vi "TryUpdateDisplacementSample.vi"   [LabVIEW 2016]
uses:
  <vilib>/rvi/DataTransferAndStorage/Container/XNode/niFpgaContainer.xnode
  <vilib>/rvi/FIFO/Fifo_Resource/nirvififoEmulationRead.vi
  <vilib>/rvi/FIFO/Fifo_Resource/nirvififoEmulationWrite.vi
  Telemetry/TelemetryDataTypes.ctl
  Telemetry/TelemetryUpdateModes.ctl
  Telemetry/TelemetryFields.ctl
  <vilib>/rvi/DataTransferAndStorage/Register/Emulation/niFpgaRegisterEmulation.vi
  <vilib>/Platform/TimedLoop/XDataNode/XDataNode.xnode
  <vilib>/Platform/TimedLoop/XDataNode/nitl_modes.ctl
  <vilib>/Platform/TimedLoop/XDataNode/XDNodeRunTimeDep.lvlib
  <vilib>/Platform/TimedLoop/XDataNode/wakeup.ctl
  <vilib>/Platform/TimedLoop/XDataNode/timing_clust.ctl
types:
  T1 = cluster{"Timestamp":u64, "TxBytes":u64, "RxBytes":u64, "TxFrames":u64, "RxFrames":u64, "Sensor1Raw":i32, "Sensor2Raw":i32, "Sensor3Raw":i32, "Sensor4Raw":i32, "Sensor5Raw":i32, "Sensor6Raw":i32, "Sensor7Raw":i32, "Sensor8Raw":i32, "Sensor1Eng":sgl, "Sensor2Eng":sgl, "Sensor3Eng":sgl, "Sensor4Eng":sgl, "Sensor5Eng":sgl, "Sensor6Eng":sgl, "Sensor7Eng":sgl, "Sensor8Eng":sgl, "PositionX":sgl, "PositionY":sgl, "PositionZ":sgl, "RotationX":sgl, "RotationY":sgl, "RotationZ":sgl}
  T2 = typedef "TelemetryFields.ctl" = enum16{"None", "InclinometerTxBytes", "InclinometerRxBytes", "InclinometerTxFrames", "InclinometerRxFrames", "InclinometerErrorTimestamp", "InclinometerErrorCode", "InclinometerSampleTimestamp", "InclinometerRawAngle", "InclinometerZenithAngle", "DisplacementTxBytes", "DisplacementRxBytes", "DisplacementTxFrames", "DisplacementRxFrames", "DisplacementErrorTimestamp", "DisplacementErrorCode", "DisplacementSampleTimestamp", "DisplacementRaw1", "DisplacementRaw2", "DisplacementRaw3", "DisplacementRaw4", "DisplacementRaw5", "DisplacementRaw6", "DisplacementRaw7", "DisplacementRaw8", "DisplacementEng1", "DisplacementEng2", "DisplacementEng3", "DisplacementEng4", "DisplacementEng5", "DisplacementEng6", "DisplacementEng7", "DisplacementEng8", "DisplacementPositionX", "DisplacementPositionY", "DisplacementPositionZ", "DisplacementRotationX", "DisplacementRotationY", "DisplacementRotationZ", "AccelerometerSampleCount", "AccelerometerSampleTimestamp", "AccelerometerRaw1", "AccelerometerRaw2", "AccelerometerRaw3", "AccelerometerRaw4", "AccelerometerRaw5", "AccelerometerRaw6", "AccelerometerRaw7", "AccelerometerRaw8", "AccelerometerEng1", "AccelerometerEng2", "AccelerometerEng3", "AccelerometerEng4", "AccelerometerEng5", "AccelerometerEng6", "AccelerometerEng7", "AccelerometerEng8", "AngularAccelerationX", "AngularAccelerationY", "AngularAccelerationZ", "GyroTxBytes", "GyroRxBytes", "GyroTxFrames", "GyroRxFrames", "GyroErrorTimestamp", "GyroErrorCode", "GyroSampleTimestamp", "GyroX", "GyroY", "GyroZ", "GyroStatus", "GyroSequenceNumber", "GyroTemperature", "GyroBITTimestamp", "GyroBIT0", "GyroBIT1", "GyroBIT2", "GyroBIT3", "GyroBIT4", "GyroBIT5", "GyroBIT6", "GyroBIT7"}
  T3 = typedef "TelemetryUpdateModes.ctl" = enum8{"=", "+", "-", "|"}
  T4 = typedef "TelemetryDataTypes.ctl" = enum8{"U8", "U16", "U32", "U64", "I8", "I16", "I32", "I64", "SGL"}
  T5 = typedef "XDNodeRunTimeDep.lvlib/timing_clust.ctl" = cluster{"Expected End [f-1]":u64, "Actual End [f-1]":u64, "Finished Late? [f-1]":bool, "Expected End [i-1]":u64, "Actual End [i-1]":u64, "Finished Late? [i-1]":bool, "Expected Start [i]":u64, "Actual Start [i]":u64, "Expected Start [f]":u64, "Actual Start [f]":u64, "Source Name":string, "Structure Name":string, "Period":i64, "Deadline":i64, "Offset":i64, "Start":i64, "Priority":i32, "Timeout":i32, "Mode":T6, "Wakeup Reason":T7, "Error":errorcluster, "Source Type":string, "Secondary Source Type":string, "Global End Time":u64, "Global Start Time":u64, "Frame Duration":u64, "Iteration Duration":u64, "Assigned CPU":i32, "I/O Scan Engine Mode":u32}
  T6 = typedef "XDNodeRunTimeDep.lvlib/nitl_modes.ctl" = enum32{"No Change", "Process missed periods, maintain original phase", "Discard missed periods, maintain original phase", "Process missed periods, ignore original phase", "Discard missed periods, ignore original phase"}
  T7 = typedef "XDNodeRunTimeDep.lvlib/wakeup.ctl" = enum32{"Normal", "Aborted", "Asynchronous wakeup", "Timing source error", "Timed loop error", "Timeout"}
  T8 = typedef "TelemetryUpdateData.ctl" = cluster{"DataType":T4, "Mode":T3, "Field":T2, "Data":u64}
  T9 = typedef "TelemetryUpdateDataSGL.ctl" = cluster{"Mode":T3, "Field":T2, "Data":sgl}
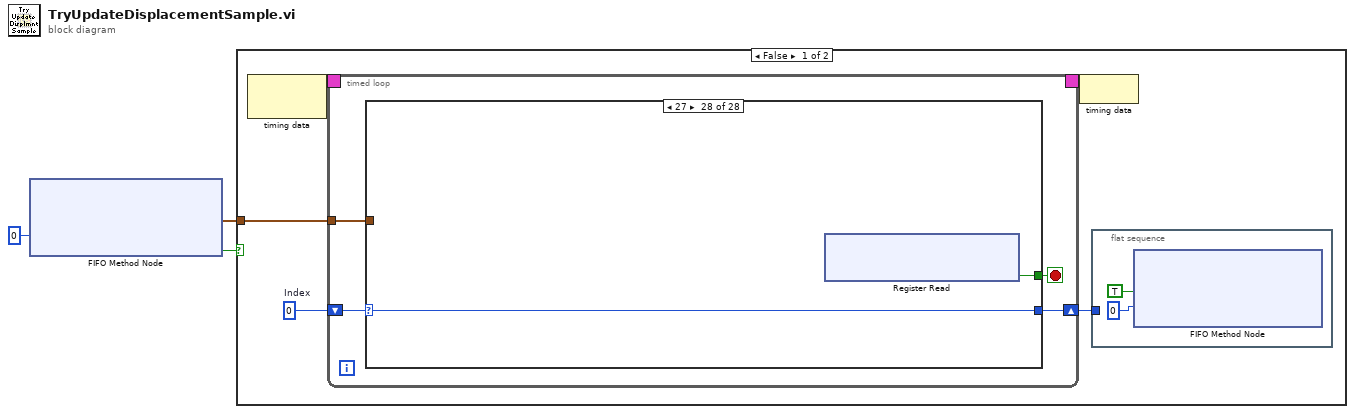
[diagram p0: block diagram]
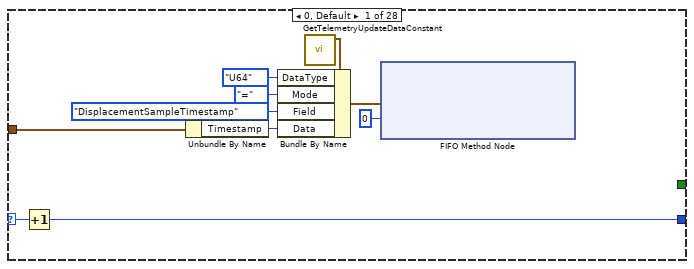
[diagram p2: hidden frame]
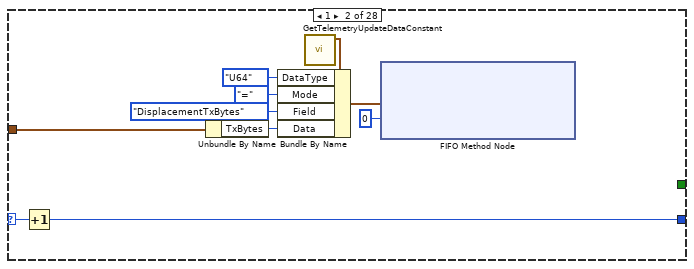
[diagram p3: hidden frame]
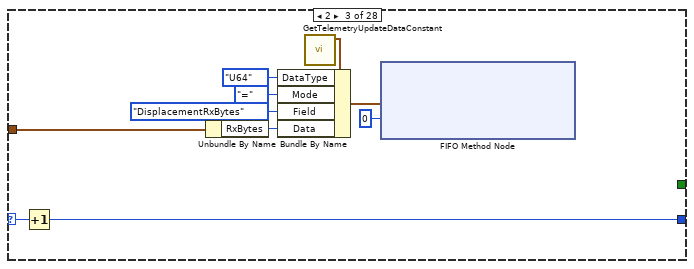
[diagram p4: hidden frame]
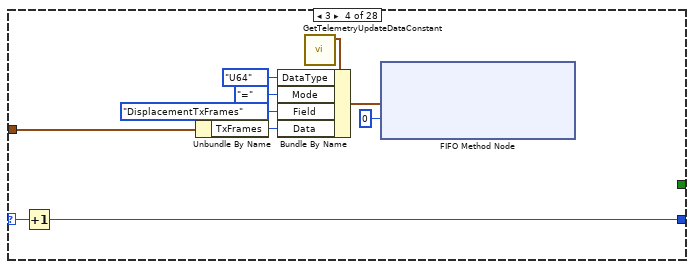
[diagram p5: hidden frame]
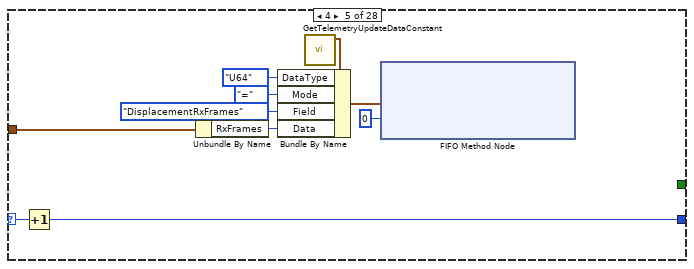
[diagram p6: hidden frame]
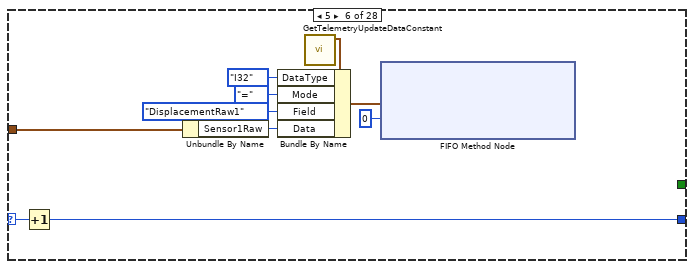
[diagram p7: hidden frame]
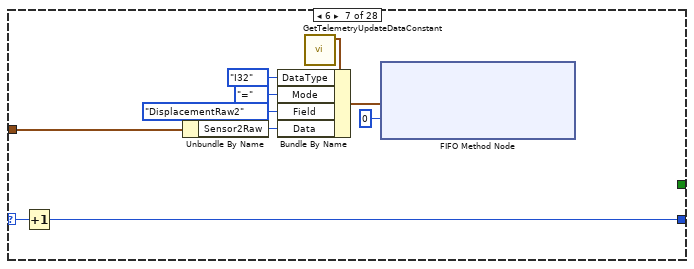
[diagram p8: hidden frame]
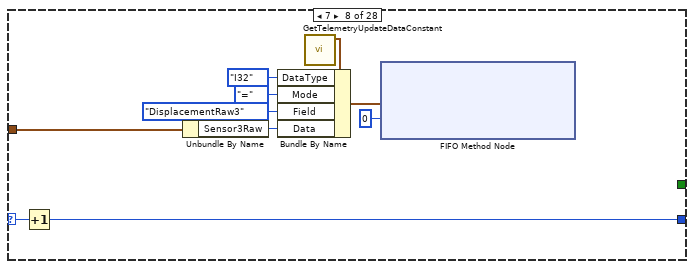
[diagram p9: hidden frame]
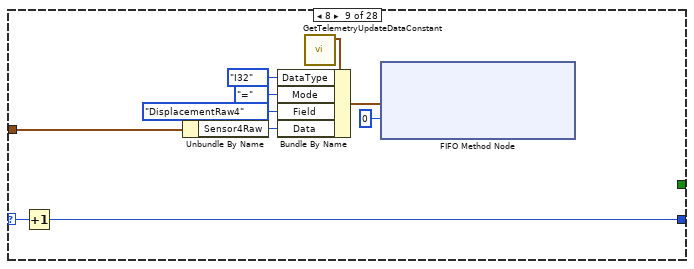
[diagram p10: hidden frame]
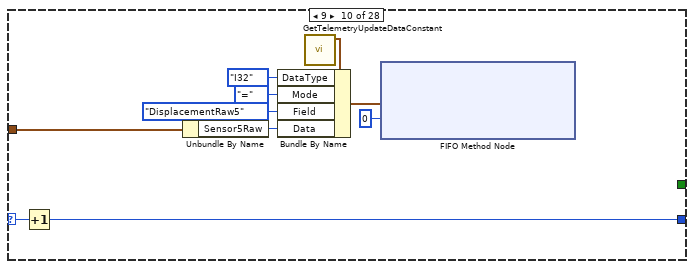
[diagram p11: hidden frame]
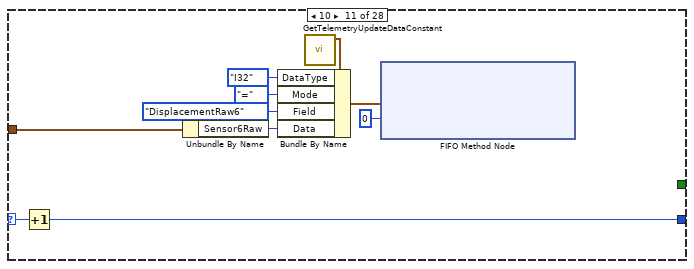
[diagram p12: hidden frame]
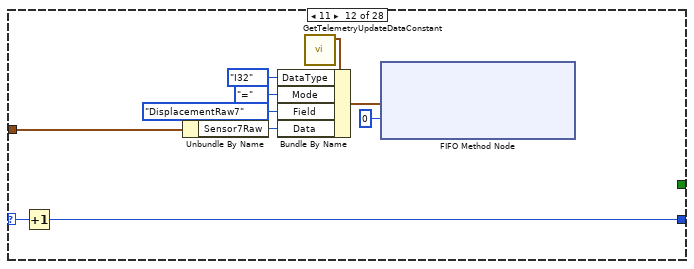
[diagram p13: hidden frame]
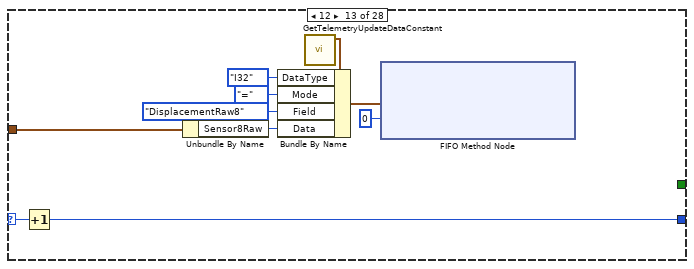
[diagram p14: hidden frame]
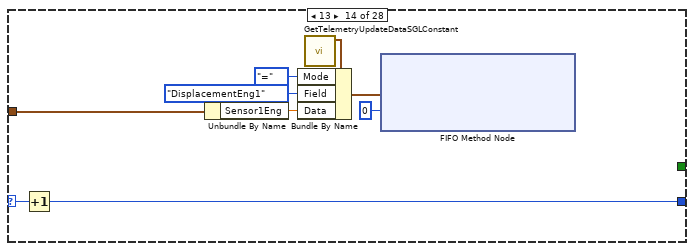
[diagram p15: hidden frame]
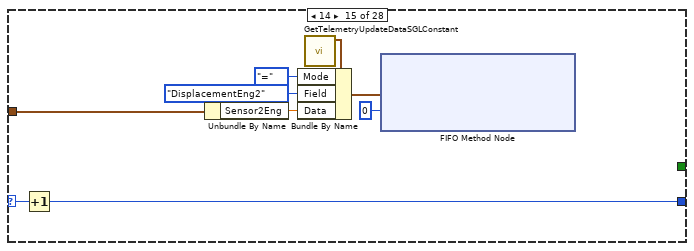
[diagram p16: hidden frame]
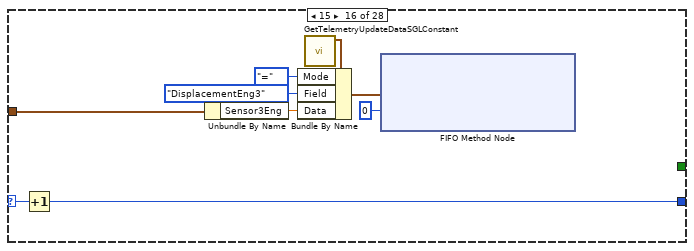
[diagram p17: hidden frame]
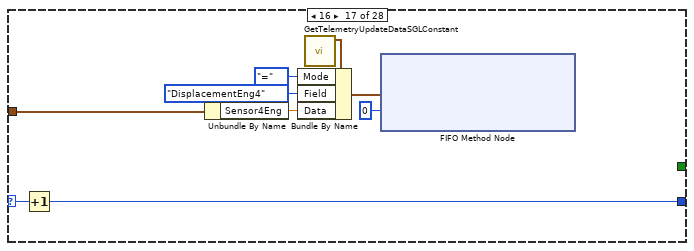
[diagram p18: hidden frame]
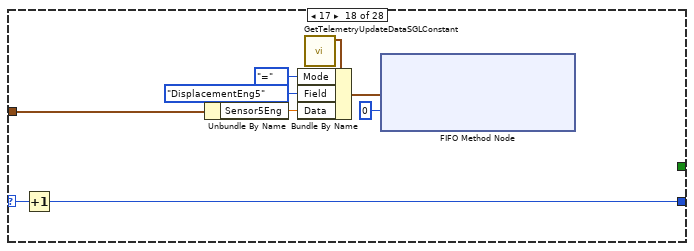
[diagram p19: hidden frame]
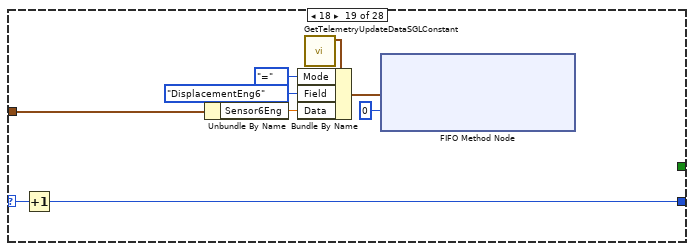
[diagram p20: hidden frame]
diagram:
  n1 = xnode ("FIFO Method Node")("Timeout"=0) -> ("Element"=w1:T1, "Timed Out?"=w2:bool)  [unwired: 1 in, 1 out]
  n2 = case shown="False" w2 {
    tunnel: w1 -> [w7 _]
    frame False {
      w8 = u8 0  # Index
      n3 = node-c288() -> (w5:T5)  [unwired: 1 in]
      n4 = timed-loop {
        shift-right: [w11] -> w6
        shift-left: w8 -> [w12]
        tunnel: w7 -> [w10]
        timing: w5 -> [_]
        timing-out: [_] -> w4
        stop <- w9 stop-if-true
        n5 = case shown="27" w12 {
          selector: w12 -> [w22 w32 w42 w52 w62 w72 w82 w92 w102 w112 w122 w132 w142 w151 w160 w169 w178 w187 w196 w205 w214 w223 w232 w241 w250 w259 w268 w270]
          tunnel: [w21 w31 w41 w51 w61 w71 w81 w91 w101 w111 w121 w131 w141 w150 w159 w168 w177 w186 w195 w204 w213 w222 w231 w240 w249 w258 w267 w270] -> w11
          tunnel: w10 -> [w13 w23 w33 w43 w53 w63 w73 w83 w93 w103 w113 w123 w133 w143 w152 w161 w170 w179 w188 w197 w206 w215 w224 w233 w242 w251 w260 _]
          tunnel: [_ _ _ _ _ _ _ _ _ _ _ _ _ _ _ _ _ _ _ _ _ _ _ _ _ _ _ w269] -> w9
          frame 0, Default {
            n6 = Increment(x=w22) -> (x+1=w21:u8)
            n7 = Unbundle By Name(w13) -> ("Timestamp"=w19:u64)
            n8 = call "GetTelemetryUpdateDataConstant.vi"() -> ("TelemetryUpdateData"=w18:T8)  [unwired: 11 in]
            n9 = Bundle By Name(cluster=w18, "DataType"=TelemetryDataTypes."U64", "Mode"=TelemetryUpdateModes."=", "Field"=TelemetryFields."DisplacementSampleTimestamp" ("TelemetryFields"), "Data"=w19) -> (w15:T8)
            n10 = xnode ("FIFO Method Node")("Element"=w15, "Timeout"=0) -> ()  [unwired: 1 in, 2 out]
          }
          frame 1 {
            n11 = Increment(x=w32) -> (x+1=w31:u8)
            n12 = Unbundle By Name(w23) -> ("TxBytes"=w24:u64)
            n13 = call "GetTelemetryUpdateDataConstant.vi"() -> ("TelemetryUpdateData"=w25:T8)  [unwired: 11 in]
            n14 = Bundle By Name(cluster=w25, "DataType"=TelemetryDataTypes."U64", "Mode"=TelemetryUpdateModes."=", "Field"=TelemetryFields."DisplacementTxBytes", "Data"=w24) -> (w29:T8)
            n15 = xnode ("FIFO Method Node")("Element"=w29, "Timeout"=0) -> ()  [unwired: 1 in, 2 out]
          }
          frame 2 {
            n16 = Increment(x=w42) -> (x+1=w41:u8)
            n17 = Unbundle By Name(w33) -> ("RxBytes"=w40:u64)
            n18 = call "GetTelemetryUpdateDataConstant.vi"() -> ("TelemetryUpdateData"=w39:T8)  [unwired: 11 in]
            n19 = Bundle By Name(cluster=w39, "DataType"=TelemetryDataTypes."U64", "Mode"=TelemetryUpdateModes."=", "Field"=TelemetryFields."DisplacementRxBytes", "Data"=w40) -> (w35:T8)
            n20 = xnode ("FIFO Method Node")("Element"=w35, "Timeout"=0) -> ()  [unwired: 1 in, 2 out]
          }
          frame 3 {
            n21 = Increment(x=w52) -> (x+1=w51:u8)
            n22 = Unbundle By Name(w43) -> ("TxFrames"=w44:u64)
            n23 = call "GetTelemetryUpdateDataConstant.vi"() -> ("TelemetryUpdateData"=w45:T8)  [unwired: 11 in]
            n24 = Bundle By Name(cluster=w45, "DataType"=TelemetryDataTypes."U64", "Mode"=TelemetryUpdateModes."=", "Field"=TelemetryFields."DisplacementTxFrames", "Data"=w44) -> (w49:T8)
            n25 = xnode ("FIFO Method Node")("Element"=w49, "Timeout"=0) -> ()  [unwired: 1 in, 2 out]
          }
          frame 4 {
            n26 = Increment(x=w62) -> (x+1=w61:u8)
            n27 = Unbundle By Name(w53) -> ("RxFrames"=w60:u64)
            n28 = call "GetTelemetryUpdateDataConstant.vi"() -> ("TelemetryUpdateData"=w59:T8)  [unwired: 11 in]
            n29 = Bundle By Name(cluster=w59, "DataType"=TelemetryDataTypes."U64", "Mode"=TelemetryUpdateModes."=", "Field"=TelemetryFields."DisplacementRxFrames", "Data"=w60) -> (w55:T8)
            n30 = xnode ("FIFO Method Node")("Element"=w55, "Timeout"=0) -> ()  [unwired: 1 in, 2 out]
          }
          frame 5 {
            n31 = Increment(x=w72) -> (x+1=w71:u8)
            n32 = Unbundle By Name(w63) -> ("Sensor1Raw"=w64:i32)
            n33 = call "GetTelemetryUpdateDataConstant.vi"() -> ("TelemetryUpdateData"=w65:T8)  [unwired: 11 in]
            n34 = Bundle By Name(cluster=w65, "DataType"=TelemetryDataTypes."I32", "Mode"=TelemetryUpdateModes."=", "Field"=TelemetryFields."DisplacementRaw1" ("TelemetryFields"), "Data"=w64) -> (w68:T8)
            n35 = xnode ("FIFO Method Node")("Element"=w68, "Timeout"=0) -> ()  [unwired: 1 in, 2 out]
          }
          frame 6 {
            n36 = Increment(x=w82) -> (x+1=w81:u8)
            n37 = Unbundle By Name(w73) -> ("Sensor2Raw"=w79:i32)
            n38 = call "GetTelemetryUpdateDataConstant.vi"() -> ("TelemetryUpdateData"=w78:T8)  [unwired: 11 in]
            n39 = Bundle By Name(cluster=w78, "DataType"=TelemetryDataTypes."I32", "Mode"=TelemetryUpdateModes."=", "Field"=TelemetryFields."DisplacementRaw2" ("TelemetryFields"), "Data"=w79) -> (w75:T8)
            n40 = xnode ("FIFO Method Node")("Element"=w75, "Timeout"=0) -> ()  [unwired: 1 in, 2 out]
          }
          frame 7 {
            n41 = Increment(x=w92) -> (x+1=w91:u8)
            n42 = Unbundle By Name(w83) -> ("Sensor3Raw"=w84:i32)
            n43 = call "GetTelemetryUpdateDataConstant.vi"() -> ("TelemetryUpdateData"=w85:T8)  [unwired: 11 in]
            n44 = Bundle By Name(cluster=w85, "DataType"=TelemetryDataTypes."I32", "Mode"=TelemetryUpdateModes."=", "Field"=TelemetryFields."DisplacementRaw3" ("TelemetryFields"), "Data"=w84) -> (w88:T8)
            n45 = xnode ("FIFO Method Node")("Element"=w88, "Timeout"=0) -> ()  [unwired: 1 in, 2 out]
          }
          frame 8 {
            n46 = Increment(x=w102) -> (x+1=w101:u8)
            n47 = Unbundle By Name(w93) -> ("Sensor4Raw"=w99:i32)
            n48 = call "GetTelemetryUpdateDataConstant.vi"() -> ("TelemetryUpdateData"=w98:T8)  [unwired: 11 in]
            n49 = Bundle By Name(cluster=w98, "DataType"=TelemetryDataTypes."I32", "Mode"=TelemetryUpdateModes."=", "Field"=TelemetryFields."DisplacementRaw4" ("TelemetryFields"), "Data"=w99) -> (w95:T8)
            n50 = xnode ("FIFO Method Node")("Element"=w95, "Timeout"=0) -> ()  [unwired: 1 in, 2 out]
          }
          frame 9 {
            n51 = Increment(x=w112) -> (x+1=w111:u8)
            n52 = Unbundle By Name(w103) -> ("Sensor5Raw"=w104:i32)
            n53 = call "GetTelemetryUpdateDataConstant.vi"() -> ("TelemetryUpdateData"=w105:T8)  [unwired: 11 in]
            n54 = Bundle By Name(cluster=w105, "DataType"=TelemetryDataTypes."I32", "Mode"=TelemetryUpdateModes."=", "Field"=TelemetryFields."DisplacementRaw5" ("TelemetryFields"), "Data"=w104) -> (w108:T8)
            n55 = xnode ("FIFO Method Node")("Element"=w108, "Timeout"=0) -> ()  [unwired: 1 in, 2 out]
          }
          frame 10 {
            n56 = Increment(x=w122) -> (x+1=w121:u8)
            n57 = Unbundle By Name(w113) -> ("Sensor6Raw"=w119:i32)
            n58 = call "GetTelemetryUpdateDataConstant.vi"() -> ("TelemetryUpdateData"=w118:T8)  [unwired: 11 in]
            n59 = Bundle By Name(cluster=w118, "DataType"=TelemetryDataTypes."I32", "Mode"=TelemetryUpdateModes."=", "Field"=TelemetryFields."DisplacementRaw6" ("TelemetryFields"), "Data"=w119) -> (w115:T8)
            n60 = xnode ("FIFO Method Node")("Element"=w115, "Timeout"=0) -> ()  [unwired: 1 in, 2 out]
          }
          frame 11 {
            n61 = Increment(x=w132) -> (x+1=w131:u8)
            n62 = Unbundle By Name(w123) -> ("Sensor7Raw"=w124:i32)
            n63 = call "GetTelemetryUpdateDataConstant.vi"() -> ("TelemetryUpdateData"=w125:T8)  [unwired: 11 in]
            n64 = Bundle By Name(cluster=w125, "DataType"=TelemetryDataTypes."I32", "Mode"=TelemetryUpdateModes."=", "Field"=TelemetryFields."DisplacementRaw7" ("TelemetryFields"), "Data"=w124) -> (w128:T8)
            n65 = xnode ("FIFO Method Node")("Element"=w128, "Timeout"=0) -> ()  [unwired: 1 in, 2 out]
          }
          frame 12 {
            n66 = Increment(x=w142) -> (x+1=w141:u8)
            n67 = Unbundle By Name(w133) -> ("Sensor8Raw"=w139:i32)
            n68 = call "GetTelemetryUpdateDataConstant.vi"() -> ("TelemetryUpdateData"=w138:T8)  [unwired: 11 in]
            n69 = Bundle By Name(cluster=w138, "DataType"=TelemetryDataTypes."I32", "Mode"=TelemetryUpdateModes."=", "Field"=TelemetryFields."DisplacementRaw8" ("TelemetryFields"), "Data"=w139) -> (w135:T8)
            n70 = xnode ("FIFO Method Node")("Element"=w135, "Timeout"=0) -> ()  [unwired: 1 in, 2 out]
          }
          frame 13 {
            n71 = Increment(x=w151) -> (x+1=w150:u8)
            n72 = Unbundle By Name(w143) -> ("Sensor1Eng"=w149:sgl)
            n73 = call "GetTelemetryUpdateDataSGLConstant.vi"() -> ("TelemetryUpdateDataSGL"=w144:T9)  [unwired: 11 in]
            n74 = Bundle By Name(cluster=w144, "Mode"=TelemetryUpdateModes."=", "Field"=TelemetryFields."DisplacementEng1", "Data"=w149) -> (w145:T9)
            n75 = xnode ("FIFO Method Node")("Element"=w145, "Timeout"=0) -> ()  [unwired: 1 in, 2 out]
          }
          frame 14 {
            n76 = Increment(x=w160) -> (x+1=w159:u8)
            n77 = Unbundle By Name(w152) -> ("Sensor2Eng"=w158:sgl)
            n78 = call "GetTelemetryUpdateDataSGLConstant.vi"() -> ("TelemetryUpdateDataSGL"=w153:T9)  [unwired: 11 in]
            n79 = Bundle By Name(cluster=w153, "Mode"=TelemetryUpdateModes."=", "Field"=TelemetryFields."DisplacementEng2", "Data"=w158) -> (w154:T9)
            n80 = xnode ("FIFO Method Node")("Element"=w154, "Timeout"=0) -> ()  [unwired: 1 in, 2 out]
          }
          frame 15 {
            n81 = Increment(x=w169) -> (x+1=w168:u8)
            n82 = Unbundle By Name(w161) -> ("Sensor3Eng"=w167:sgl)
            n83 = call "GetTelemetryUpdateDataSGLConstant.vi"() -> ("TelemetryUpdateDataSGL"=w162:T9)  [unwired: 11 in]
            n84 = Bundle By Name(cluster=w162, "Mode"=TelemetryUpdateModes."=", "Field"=TelemetryFields."DisplacementEng3", "Data"=w167) -> (w163:T9)
            n85 = xnode ("FIFO Method Node")("Element"=w163, "Timeout"=0) -> ()  [unwired: 1 in, 2 out]
          }
          frame 16 {
            n86 = Increment(x=w178) -> (x+1=w177:u8)
            n87 = Unbundle By Name(w170) -> ("Sensor4Eng"=w176:sgl)
            n88 = call "GetTelemetryUpdateDataSGLConstant.vi"() -> ("TelemetryUpdateDataSGL"=w171:T9)  [unwired: 11 in]
            n89 = Bundle By Name(cluster=w171, "Mode"=TelemetryUpdateModes."=", "Field"=TelemetryFields."DisplacementEng4", "Data"=w176) -> (w172:T9)
            n90 = xnode ("FIFO Method Node")("Element"=w172, "Timeout"=0) -> ()  [unwired: 1 in, 2 out]
          }
          frame 17 {
            n91 = Increment(x=w187) -> (x+1=w186:u8)
            n92 = Unbundle By Name(w179) -> ("Sensor5Eng"=w185:sgl)
            n93 = call "GetTelemetryUpdateDataSGLConstant.vi"() -> ("TelemetryUpdateDataSGL"=w180:T9)  [unwired: 11 in]
            n94 = Bundle By Name(cluster=w180, "Mode"=TelemetryUpdateModes."=", "Field"=TelemetryFields."DisplacementEng5", "Data"=w185) -> (w181:T9)
            n95 = xnode ("FIFO Method Node")("Element"=w181, "Timeout"=0) -> ()  [unwired: 1 in, 2 out]
          }
          frame 18 {
            n96 = Increment(x=w196) -> (x+1=w195:u8)
            n97 = Unbundle By Name(w188) -> ("Sensor6Eng"=w194:sgl)
            n98 = call "GetTelemetryUpdateDataSGLConstant.vi"() -> ("TelemetryUpdateDataSGL"=w189:T9)  [unwired: 11 in]
            n99 = Bundle By Name(cluster=w189, "Mode"=TelemetryUpdateModes."=", "Field"=TelemetryFields."DisplacementEng6", "Data"=w194) -> (w190:T9)
            n100 = xnode ("FIFO Method Node")("Element"=w190, "Timeout"=0) -> ()  [unwired: 1 in, 2 out]
          }
          frame 19 {
            n101 = Increment(x=w205) -> (x+1=w204:u8)
            n102 = Unbundle By Name(w197) -> ("Sensor7Eng"=w203:sgl)
            n103 = call "GetTelemetryUpdateDataSGLConstant.vi"() -> ("TelemetryUpdateDataSGL"=w198:T9)  [unwired: 11 in]
            n104 = Bundle By Name(cluster=w198, "Mode"=TelemetryUpdateModes."=", "Field"=TelemetryFields."DisplacementEng7", "Data"=w203) -> (w199:T9)
            n105 = xnode ("FIFO Method Node")("Element"=w199, "Timeout"=0) -> ()  [unwired: 1 in, 2 out]
          }
          frame 20 {
            n106 = Increment(x=w214) -> (x+1=w213:u8)
            n107 = Unbundle By Name(w206) -> ("Sensor8Eng"=w212:sgl)
            n108 = call "GetTelemetryUpdateDataSGLConstant.vi"() -> ("TelemetryUpdateDataSGL"=w207:T9)  [unwired: 11 in]
            n109 = Bundle By Name(cluster=w207, "Mode"=TelemetryUpdateModes."=", "Field"=TelemetryFields."DisplacementEng8", "Data"=w212) -> (w208:T9)
            n110 = xnode ("FIFO Method Node")("Element"=w208, "Timeout"=0) -> ()  [unwired: 1 in, 2 out]
          }
          frame 21 {
            n111 = Increment(x=w223) -> (x+1=w222:u8)
            n112 = Unbundle By Name(w215) -> ("PositionX"=w221:sgl)
            n113 = call "GetTelemetryUpdateDataSGLConstant.vi"() -> ("TelemetryUpdateDataSGL"=w216:T9)  [unwired: 11 in]
            n114 = Bundle By Name(cluster=w216, "Mode"=TelemetryUpdateModes."=", "Field"=TelemetryFields."DisplacementPositionX", "Data"=w221) -> (w217:T9)
            n115 = xnode ("FIFO Method Node")("Element"=w217, "Timeout"=0) -> ()  [unwired: 1 in, 2 out]
          }
          frame 22 {
            n116 = Increment(x=w232) -> (x+1=w231:u8)
            n117 = Unbundle By Name(w224) -> ("PositionY"=w230:sgl)
            n118 = call "GetTelemetryUpdateDataSGLConstant.vi"() -> ("TelemetryUpdateDataSGL"=w225:T9)  [unwired: 11 in]
            n119 = Bundle By Name(cluster=w225, "Mode"=TelemetryUpdateModes."=", "Field"=TelemetryFields."DisplacementPositionY", "Data"=w230) -> (w226:T9)
            n120 = xnode ("FIFO Method Node")("Element"=w226, "Timeout"=0) -> ()  [unwired: 1 in, 2 out]
          }
          frame 23 {
            n121 = Increment(x=w241) -> (x+1=w240:u8)
            n122 = Unbundle By Name(w233) -> ("PositionZ"=w239:sgl)
            n123 = call "GetTelemetryUpdateDataSGLConstant.vi"() -> ("TelemetryUpdateDataSGL"=w234:T9)  [unwired: 11 in]
            n124 = Bundle By Name(cluster=w234, "Mode"=TelemetryUpdateModes."=", "Field"=TelemetryFields."DisplacementPositionZ", "Data"=w239) -> (w235:T9)
            n125 = xnode ("FIFO Method Node")("Element"=w235, "Timeout"=0) -> ()  [unwired: 1 in, 2 out]
          }
          frame 24 {
            n126 = Increment(x=w250) -> (x+1=w249:u8)
            n127 = Unbundle By Name(w242) -> ("RotationX"=w248:sgl)
            n128 = call "GetTelemetryUpdateDataSGLConstant.vi"() -> ("TelemetryUpdateDataSGL"=w243:T9)  [unwired: 11 in]
            n129 = Bundle By Name(cluster=w243, "Mode"=TelemetryUpdateModes."=", "Field"=TelemetryFields."DisplacementRotationX", "Data"=w248) -> (w244:T9)
            n130 = xnode ("FIFO Method Node")("Element"=w244, "Timeout"=0) -> ()  [unwired: 1 in, 2 out]
          }
          frame 25 {
            n131 = Increment(x=w259) -> (x+1=w258:u8)
            n132 = Unbundle By Name(w251) -> ("RotationY"=w257:sgl)
            n133 = call "GetTelemetryUpdateDataSGLConstant.vi"() -> ("TelemetryUpdateDataSGL"=w252:T9)  [unwired: 11 in]
            n134 = Bundle By Name(cluster=w252, "Mode"=TelemetryUpdateModes."=", "Field"=TelemetryFields."DisplacementRotationY", "Data"=w257) -> (w253:T9)
            n135 = xnode ("FIFO Method Node")("Element"=w253, "Timeout"=0) -> ()  [unwired: 1 in, 2 out]
          }
          frame 26 {
            n136 = Increment(x=w268) -> (x+1=w267:u8)
            n137 = Unbundle By Name(w260) -> ("RotationZ"=w266:sgl)
            n138 = call "GetTelemetryUpdateDataSGLConstant.vi"() -> ("TelemetryUpdateDataSGL"=w261:T9)  [unwired: 11 in]
            n139 = Bundle By Name(cluster=w261, "Mode"=TelemetryUpdateModes."=", "Field"=TelemetryFields."DisplacementRotationZ", "Data"=w266) -> (w262:T9)
            n140 = xnode ("FIFO Method Node")("Element"=w262, "Timeout"=0) -> ()  [unwired: 1 in, 2 out]
          }
          frame 27 {
            n141 = xnode ("Register Read")() -> ("Data"=w269:bool)  [unwired: 1 in, 1 out]
          }
        }
      }
      n142 = node-c288(w4) -> ()
      n143 = flat-sequence {
        tunnel: w6 -> [_]
        frame #0 {
          n144 = xnode ("FIFO Method Node")("Element"=TRUE, "Timeout"=0) -> ()  [unwired: 1 in, 2 out]
        }
      }
    }
    frame True {
    }
  }
